vi "CreateSpectrum.vi"(8 "error in (no error)":errorcluster, 10 "Lambda max":dbl=780.0 format="%#_13g", 11 "Lambda min":dbl=440.0 format="%#_13g") -> (0 "error out":errorcluster, 3 "Color Ramp (zero is black)":u32[](array[colorbox]))   [LabVIEW 2023]
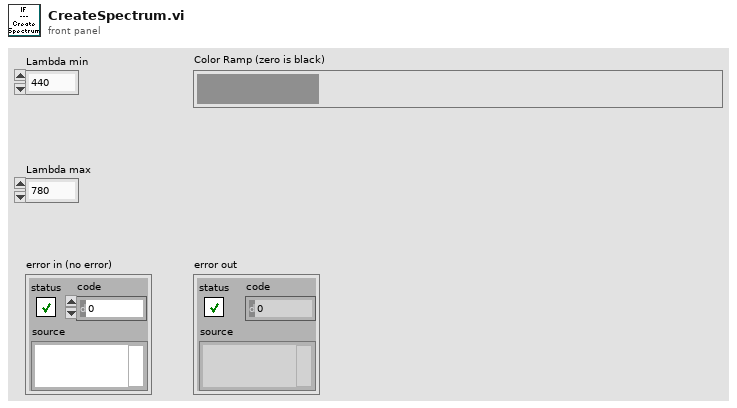
[diagram p1: front panel]
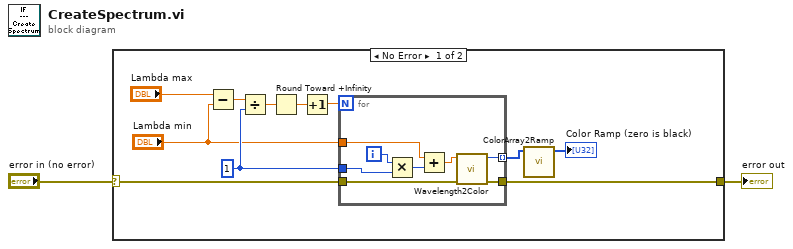
[diagram p0: block diagram]
diagram:
  n1 = case shown="No Error" "error in (no error)" {
    selector: "error in (no error)" -> [w13 w22]
    tunnel: [w12 w22] -> w2
    frame No Error {
      w6 = u8 1 ("Sparse factor")
      n2 = Subtract(x="Lambda max", y="Lambda min") -> (x-y=w11:dbl)
      n3 = Divide(x=w11, y=w6) -> (x/y=w10:dbl)
      n4 = Round Toward +Infinity(x=w10) -> (ceil(x): smallest int >= x=w9:dbl)
      n5 = Increment(x=w9) -> (x+1=w8:dbl)
      n6 = for {
        N: w8 -> [_]
        tunnel: "Lambda min" -> [w21]
        tunnel: [w19] -> w7 mode=indexing
        tunnel: w13 -> [w18]
        tunnel: [w17] -> w12
        tunnel: w6 -> [w14]
        i -> [w15]
        n7 = Multiply(x=w15, y=w14) -> (x*y=w16:i32)
        n8 = Add(x=w21, y=w16) -> (x+y=w20:dbl)
        n9 = call "Wavelength2Color.vi"("error in (no error)"=w18, "Wavelength"=w20) -> ("error out"=w17:errorcluster, "Color"=w19:u32)  [unwired: 8 in]
      }
      n10 = call "ColorArray2Ramp.vi"("Color Array"=w7) -> ("Color Ramp (zero is black)"=→"Color Ramp (zero is black)":u32[])  [unwired: 10 in]
    }
    frame Error {
    }
  }
  "error out" <- w2
